vi "2D Array Min Max.vi"(2 "Rows Include":i32, 3 "Array":dbl[][](array[numeric])) -> (0 "min value":dbl, 1 "max value":dbl)   [LabVIEW 2017, in "Measurement.PhotocurrentMapping.UI.lvclass"]
uses:
  Measurement.PhotocurrentMapping.UI.lvclass
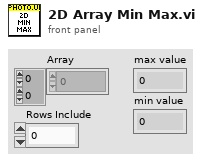
[diagram p1: front panel]
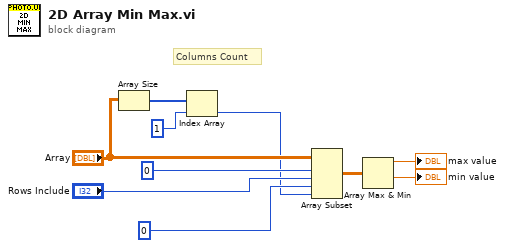
[diagram p0: block diagram]
diagram:
  # "Columns Count"
  n1 = Array Size(array="Array") -> (size(s)=w10:i32[])
  n2 = Index Array(array=w10, index=1) -> (element=w4:i32)
  n3 = Array Subset(array="Array", index (row)=0 ("index"), length (row)="Rows Include", index (col)=0 ("index"), length (col)=w4) -> (w3:dbl[][])
  n4 = Array Max & Min(array=w3) -> (max value=→"max value":dbl, min value=→"min value":dbl)  [unwired: 2 out]
